vi "split magnet graph into 3.vi"(10 "graph in":cluster{sgl[], sgl[]}) -> (2 "graph array":cluster{sgl[], sgl[]}[](array[cluster]))   [LabVIEW 2017]
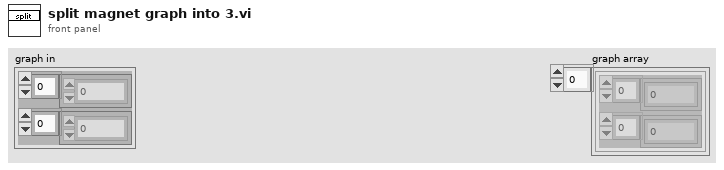
[diagram p1: front panel]
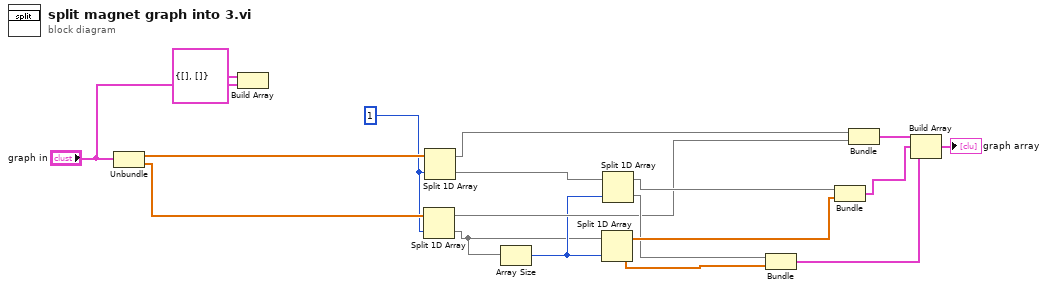
[diagram p0: block diagram]
diagram:
  w5 = 1 ("index")
  n1 = Unbundle("graph in") -> (w18:sgl[], w17:sgl[])
  n2 = Build Array(cluster{sgl[], sgl[]} {[], []} ("element"), "graph in") -> ()  [unwired: 1 out]
  n3 = Split 1D Array(array=w17, index=w5) -> (first subarray=w4:sgl[], second subarray=w1:sgl[])
  n4 = Split 1D Array(array=w18, index=w5) -> (first subarray=w15:sgl[], second subarray=w16:sgl[])
  n5 = Array Size(array=w1) -> (size(s)=w3:i32)
  n6 = Split 1D Array(array=w1, index=w3) -> (first subarray=w13:sgl[], second subarray=w11:sgl[])
  n7 = Split 1D Array(array=w16, index=w3) -> (first subarray=w14:sgl[], second subarray=w12:sgl[])
  n8 = Bundle(w12, w11) -> (w8:cluster{sgl[], sgl[]})  [unwired: 1 in]
  n9 = Bundle(w14, w13) -> (w9:cluster{sgl[], sgl[]})  [unwired: 1 in]
  n10 = Bundle(w15, w4) -> (w10:cluster{sgl[], sgl[]})  [unwired: 1 in]
  n11 = Build Array(w10, w9, w8) -> (→"graph array":cluster{sgl[], sgl[]}[])
